vi "Read Actor List.vi"(8 "error in (no error)":errorcluster, 11 "CS++ObjectManager in":refnum<class "CS++ObjectManager.lvclass">) -> (0 "error out":errorcluster, 3 "CS++ObjectManager out":refnum<class "CS++ObjectManager.lvclass">)   [LabVIEW 2016, in "CS++ObjectManager.lvlib" / "CS++ObjectManager.lvclass"]
doc: "Read Actor List from DB Connection."
uses:
  CS++ObjectManager.lvclass
  C:/User/Brand/LVP/TASCA/UTCS/Packages/CSPP_Core/Actors/CS++BaseActor/CS++BaseActor.lvclass
  CSPP_Core/Actors/CS++BaseActor/CS++BaseActor.lvclass/CS++BaseActor.ctl
  CS++ObjectManager.lvclass/CS++ObjectManager.ctl
  CSPP_Core/Classes/CS++BaseClasses/Factory/CS++Factory.lvclass
  CSPP_Core/Libraries/Utilities/CS++Utilities.lvlib
  CSPP_Core/Actors/CS++BaseActor/CS++BaseActor.lvclass
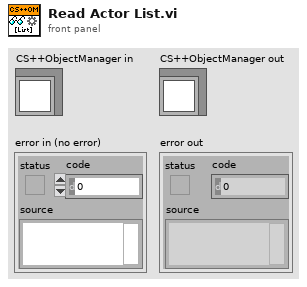
[diagram p1: front panel]
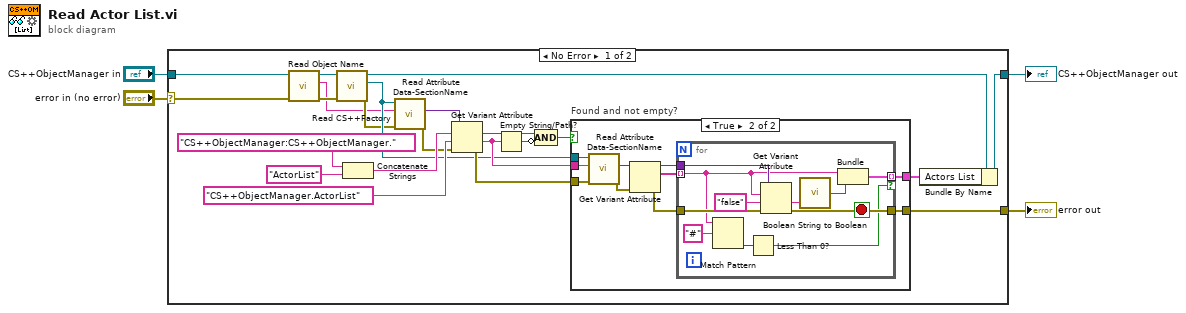
[diagram p0: block diagram]
diagram:
  n1 = case shown="No Error" "error in (no error)" {
    selector: "error in (no error)" -> [w14 w50]
    tunnel: [w17 w50] -> w1
    tunnel: [w19 w49] -> w2
    tunnel: "CS++ObjectManager in" -> [w16 w49]
    frame No Error {
      n2 = call "Read Object Name.vi"("error in (no error)"=w14, "CS++BaseActor in"=w16) -> ("error out"=w13:errorcluster, "Object Name"=w5:string, "CS++BaseActor out"=w15:refnum<class "CS++ObjectManager.lvclass">)  [unwired: 7 in]
      n3 = call "Read CS++Factory.vi"("error in (no error)"=w13, "CS++BaseActor in"=w15) -> ("error out"=w6:errorcluster, "CS++Factory"=w7:refnum<class "CS++Factory.lvclass">, "CS++BaseActor out"=w20:refnum<class "CS++ObjectManager.lvclass">)  [unwired: 7 in]
      n4 = Concatenate Strings("CS++ObjectManager:CS++ObjectManager.", "ActorList" ("string")) -> (w12:string)
      n5 = call-dynamic "Read Attribute Data-SectionName.vi"("error in (no error)"=w6, "Object Name"=w5, "CS++Factory in"=w7) -> ("error out"=w9:errorcluster, "Attribute Data"=w8:variant)  [unwired: 6 in, 1 out]
      n6 = Get Variant Attribute(Variant=w8, name=w12, default value (empty Variant)="CS++ObjectManager.ActorList" ("string"), error in=w9) -> (found=w26:bool, value=w23:string, error out=w24:errorcluster)  [unwired: 1 out]
      n7 = Empty String/Path?(string/path=w23) -> (empty?=w25:bool)
      n8 = Compound Arithmetic op=AND(w26, invert w25) -> (w22:bool)
      n9 = case "Found and not empty?" shown="True" w22 {
        tunnel: [_ w34] -> w18
        tunnel: [w27 w33] -> w17
        tunnel: w7 -> [_ w31]
        tunnel: w24 -> [w27 w30]
        tunnel: w23 -> [_ w32]
        frame False {
        }
        frame True {
          n10 = call-dynamic "Read Attribute Data-SectionName.vi"("error in (no error)"=w30, "Object Name"=w32, "CS++Factory in"=w31) -> ("error out"=w29:errorcluster, "Attribute Data"=w28:variant)  [unwired: 6 in, 1 out]
          n11 = Get Variant Attribute(Variant=w28, error in=w29) -> (duplicate Variant=w36:variant, names=w35:string[], error out=w37:errorcluster)  [unwired: 2 in, 1 out]
          n12 = for {
            tunnel: w35 -> [w43] mode=indexing
            tunnel: [w45] -> w34 mode=indexing if=w44
            tunnel: w36 -> [w48]
            tunnel: w37 -> [w47]
            tunnel: [w46] -> w33
            stop <- w46 stop-if-true
            n13 = Match Pattern(string=w43, regular expression="#") -> (offset past match=w38:i32)  [unwired: 1 in, 3 out]
            n14 = Less Than 0?(x=w38) -> (x < 0?=w44:bool)
            n15 = Get Variant Attribute(Variant=w48, name=w43, default value (empty Variant)="false" ("string"), error in=w47) -> (value=w41:string, error out=w46:errorcluster)  [unwired: 2 out]
            n16 = call "Boolean String to Boolean.vi"("T/F String"=w41) -> ("Value"=w40:bool)
            n17 = Bundle(w43, "Value"=w40) -> (w45:cluster{string, "Value":bool})  [unwired: 1 in]
          }
        }
      }
      n18 = Bundle By Name(cluster=w20, "Actors List"=w18) -> (w19:refnum<class "CS++ObjectManager.lvclass">)
    }
    frame Error {
    }
  }
  "error out" <- w1
  "CS++ObjectManager out" <- w2
